vi "PH_PLH-AccessInformation.read DB.vi"(0 "i ref in":refnum<vi>, 5 "error in (no error)":errorcluster) -> (14 "i ref out":refnum<vi>, 19 "error out":errorcluster)   [LabVIEW 2009]
doc: "This VI reads the database entries and stores the information to own attributes."
uses:
  PH_PLH-AccessInformation.lvlib
  CSCore/BaseProcess/BaseProcess.lvlib
  PH_Common/Ctrls/Enabling State.ctl
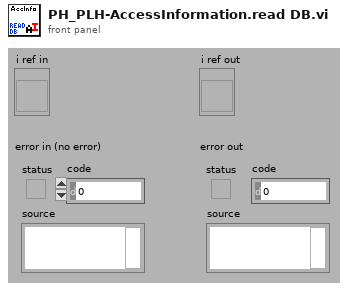
[diagram p1: front panel]
types:
  T1 = typedef "PH_PLH-AccessInformation.lvlib/PH_PLH-AccessInformation.i attribute.ctl" = cluster{"GUI Refs":cluster{"Ref Shotmode":refnum<vi>, "Ref Searchmode":refnum<vi>}, "Shotmode":i32, "Searchmode":i32}
  T2 = typedef "Enabling State.ctl" = i32
  T3 = typedef "BaseProcess.lvlib/BaseProcess.i attribute.ctl" = cluster{"EventStatus":string, "EventError":i32, "PresetEvtWatchD":i32, "PresetPdcWatchD":i32, "EventTimeout":i32, "PeriodicInterval":i32, "Interface":string[], "Address":string[], "Special":string[], "PeriodicError":i32, "PeriodicStatus":string, "SuperProc":string, "Descriptors":T4[], "CaseRef":refnum<vi>, "PdcRef":refnum<vi>, "Thread Ref":refnum<vi>, "eventErrorID":i32, "eventStatusID":i32, "periodicErrorID":i32, "periodicStatusID":i32, "pdcCtrID":i32}
  T4 = typedef "BaseProcess.lvlib/BaseProcess.descriptor definition.ctl" = cluster{"selector":string, "descriptor":T5}
  T5 = typedef "BaseProcess.lvlib/BaseProcess.descriptor string definition.ctl" = string
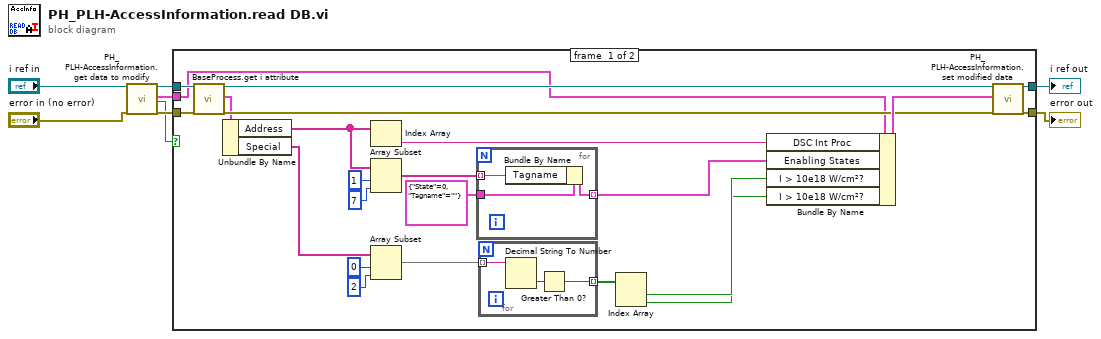
[diagram p0: block diagram]
diagram:
  n1 = call "PH_PLH-AccessInformation.get data to modify.vi"("i ref in"="i ref in", "error in (no error)"="error in (no error)") -> ("i ref out"=w6:refnum<vi>, "i attribute"=w8:T1, "timed out"=w1:bool, "error out"=w3:errorcluster)  [unwired: 14 in]
  n2 = case shown="False" w1 {
    tunnel: w6 -> [w25 w39]
    tunnel: [w31 w39] -> w4
    tunnel: w3 -> [w24 w38]
    tunnel: [w30 w38] -> w2
    tunnel: w8 -> [w22 _]
    frame #0 {
      n3 = call "BaseProcess.get i attribute.vi"("i ref in"=w25, "error in (no error)"=w24) -> ("i ref out"=w27:refnum<vi>, "i attribute"=w26:T3, "error out"=w28:errorcluster)  [unwired: 15 in]
      n4 = Unbundle By Name(w26) -> ("Address"=w19:string[], "Special"=w13:string[])
      n5 = Index Array(array=w19) -> (element=w23:string)  [unwired: 1 in]
      n6 = Array Subset(array=w19, index=1, length=7) -> (w16:string[])
      n7 = Array Subset(array=w13, index=0, length=2) -> (w12:string[])
      n8 = for {
        tunnel: cluster{"State":T2, "Tagname":string} {"State"=0, "Tagname"=""} ("State") -> [w37]
        tunnel: w16 -> [w36] mode=indexing
        tunnel: [w35] -> w21 mode=indexing
        n9 = Bundle By Name(cluster=w37, "Tagname"=w36) -> (w35:cluster{"State":T2, "Tagname":string})
      }
      n10 = for {
        tunnel: w12 -> [w33] mode=indexing
        tunnel: [w32] -> w11 mode=indexing
        n11 = Decimal String To Number(string=w33) -> (number=w34:i32)  [unwired: 2 in, 1 out]
        n12 = Greater Than 0?(x=w34) -> (x > 0?=w32:bool)
      }
      n13 = Index Array(array=w11) -> (element #1=w10:bool, element #2=w9:bool)  [unwired: 2 in]
      n14 = Bundle By Name(cluster=w22, "DSC Int Proc"=w23, "Enabling States"=w21, "I > 10e18 W/cm²?"=w10, "I > 10e18 W/cm²?"=w9) -> (w29:T1)
      n15 = call "PH_PLH-AccessInformation.set modified data.vi"("i ref in"=w27, "i attribute"=w29, "error in (no error)"=w28) -> ("i ref out"=w31:refnum<vi>, "error out"=w30:errorcluster)  [unwired: 15 in]
    }
    frame #1 {
    }
  }
  "i ref out" <- w4
  "error out" <- w2
